vi "PH_Sixpack_Switch.PC Write PSDB.vi"(0 "i ref in":refnum<vi>, 5 "error IO":errorcluster) -> (14 "i ref out":refnum<vi>, 19 "error out":errorcluster)   [LabVIEW 2014, in "PH_Sixpack_Switch.lvlib"]
doc: "This is the proc case which writes data to the PHELIX shot data base."
uses:
  PH_Sixpack_Switch.lvlib
  PH_Basics/PH_PSDBWriter/PH_PSDBWriter.lvlib
  PH_Basics/PH_AxisGUI_BaseClass/PH_AxisGUI_BaseClass.lvlib
  PH_Basics/PH_StatusHandler/PH_StatusHandler.lvlib
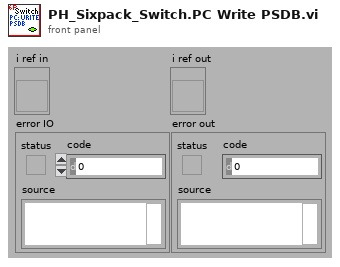
[diagram p1: front panel]
types:
  T1 = typedef "PH_AxisGUI_BaseClass.lvlib/PH_AxisGUI_BaseClass.i attribute.ctl" = cluster{"Axes":T2[]}
  T2 = typedef "PH_AxisGUI_BaseClass.lvlib/PH_AxisGUI_BaseClass.Axis Attributes.ctl" = cluster{"Axis GUI Refs":T3, "Address":T4, "Name":string, "Label \"Back\"":string, "Labell \"Forth\"":string, "Moving?":bool}
  T3 = typedef "PH_AxisGUI_BaseClass.lvlib/PH_AxisGUI_BaseClass.Axis GUI Refs.ctl" = cluster{"Back":refnum<vi>, "Forth":refnum<vi>, "Status":refnum<vi>, "Target":refnum<vi>, "Address":refnum<vi>, "Status Bar":refnum<vi>, "Settings":refnum<vi>, "Activity":refnum<vi>, "Clear Error":refnum<vi>}
  T4 = typedef "PH_Stepmotor_BaseClass.lvlib/PH_Stepmotor_BaseClass.Axis Address.ctl" = cluster{"Instance":string, "Motor Nr":i32}
  T5 = typedef "PH_PSDBWriter.lvlib/PH_PSDBWriter.String dataset.ctl" = cluster{"name":string, "data":string, "unit":string}
  T6 = typedef "PH_PSDBWriter.lvlib/PH_PSDBWriter.PSDB Dataset.ctl" = cluster{"Version":i32, "2D data Input":T7[], "Boolean Input":T9[], "Image Input":T10[], "Numeric Input":T12[], "String Input":T5[]}
  T7 = typedef "PH_PSDBWriter.lvlib/PH_PSDBWriter.2D dataset.ctl" = cluster{"name":string, "data":dbl[][], "axis description":T8}
  T8 = typedef "PSDB.lvlib/PSDB_AxisDescription.ctl" = cluster{"x axis label":string, "y axis label":string, "x axis unit":string, "y axis unit":string}
  T9 = typedef "PH_PSDBWriter.lvlib/PH_PSDBWriter.Boolean dataset.ctl" = cluster{"name":string, "data":bool, "unit":string}
  T10 = typedef "PH_PSDBWriter.lvlib/PH_PSDBWriter.Image dataset.ctl" = cluster{"name":string, "data":T11, "unit":string}
  T11 = typedef "IMAQ Image.ctl" = refnum<image>
  T12 = typedef "PH_PSDBWriter.lvlib/PH_PSDBWriter.Numeric dataset.ctl" = cluster{"name":string, "data":dbl, "unit":string}
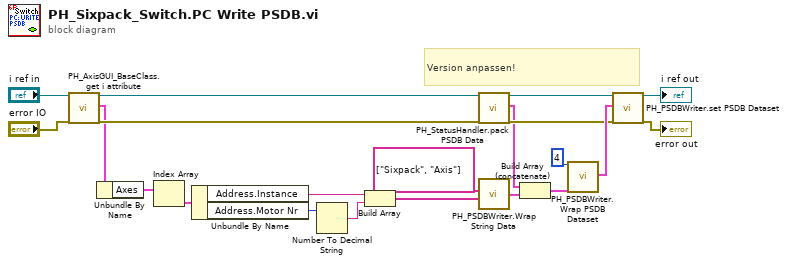
[diagram p0: block diagram]
diagram:
  # "Version anpassen!"
  n1 = call "PH_AxisGUI_BaseClass.get i attribute.vi"("i ref in"="i ref in", "error in (no error)"="error IO") -> ("i ref out"=w8:refnum<vi>, "i attribute"=w7:T1, "error out"=w10:errorcluster)  [unwired: 15 in]
  n2 = Unbundle By Name(w7) -> ("Axes"=w3:T2[])
  n3 = Index Array(array=w3) -> (element=w4:T2)  [unwired: 1 in]
  n4 = Unbundle By Name(w4) -> ("Address.Instance"=w6:string, "Address.Motor Nr"=w5:i32)
  n5 = Number To Decimal String(number=w5) -> (decimal integer string=w20:string)  [unwired: 1 in]
  n6 = Build Array(w6, w20) -> (w13:string[])
  n7 = call "PH_StatusHandler.pack PSDB Data.vi"("VI in"=w8, "error in (no error)"=w10) -> ("VI out"=w18:refnum<vi>, "PSDB String Data Array"=w1:T5[], "error out"=w11:errorcluster)  [unwired: 15 in]
  n8 = call "PH_PSDBWriter.Wrap String Data.vi"("Data Array"=w13, "Name Array"=string[] ["Sixpack", "Axis"]) -> ("PSDB String Data Array"=w12:T5[])  [unwired: 2 in]
  n9 = Build Array (concatenate)(w1, w12) -> (w2:T5[])
  n10 = call "PH_PSDBWriter.Wrap PSDB Dataset.vi"("Version"=4, "String Input"=w2) -> ("PSDB Dataset"=w16:T6)  [unwired: 17 in]
  n11 = call "PH_PSDBWriter.set PSDB Dataset.vi"("VI in"=w18, "PSDB Dataset"=w16, "error in (no error)"=w11) -> ("VI out"=→"i ref out":refnum<vi>, "error out"=→"error out":errorcluster)  [unwired: 15 in]
